vi "JKI SM EDITOR - quick filter list.vi"(0 "quick filter text":string, 1 "Num Event Frames":i32, 7 "States":string[](array[string]), 11 "error in":errorcluster) -> (6 "All Items Filtered Out":bool, 8 "States quick-filtered":string[](array[string]), 10 "Indices quick-filtered":i32[](array[numeric]), 15 "error out":errorcluster)   [LabVIEW 2013]
uses:
  JKI State Machine API/source/JKI SM/JKI SM.lvclass
panel:
  # "Copyright © 2006 James Kring, Inc. All rights reserved.\nMichael Aivaliotis michael.aivaliotis@jameskring.com\nalternate email: michael@aivaliotis.com\n\nThis library is provided \"AS IS\" , WITHOUT WARRANTIES OR \nCONDITIONS OF ANY KIND, either express or implied.\n\nJames Kring, Inc. -- http://www.jameskring.com"
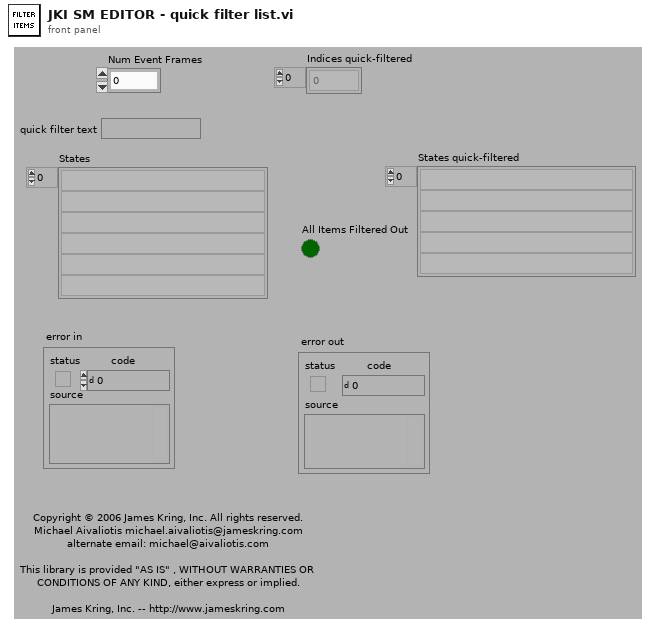
[diagram p1: front panel]
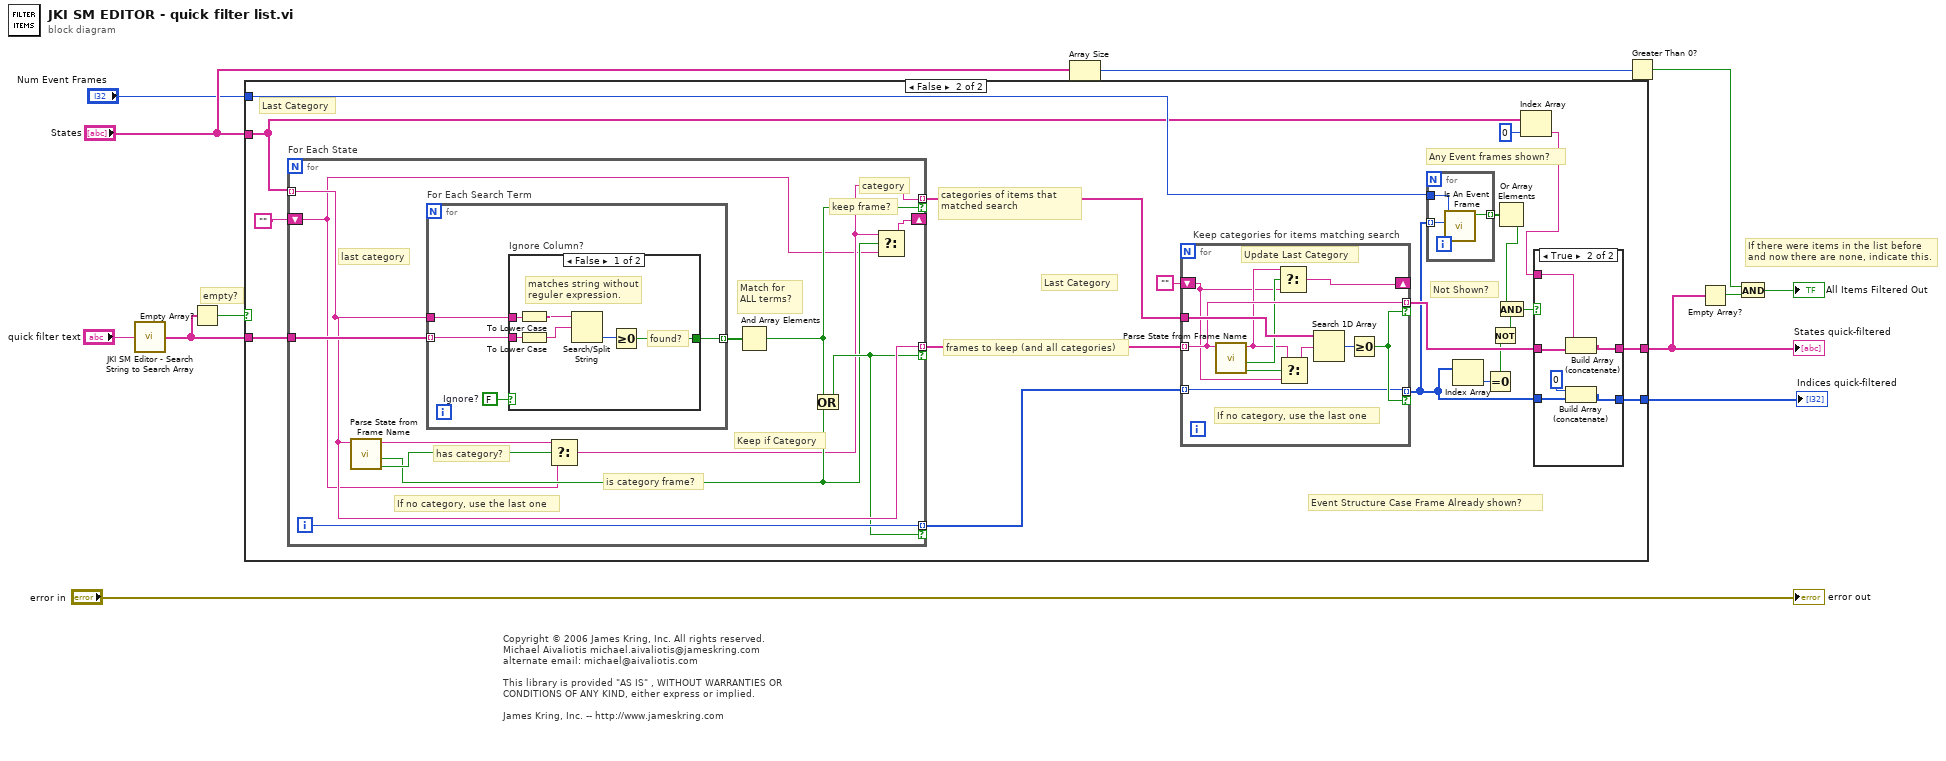
[diagram p0: block diagram]
diagram:
  # "If there were items in the list before and now there are none, indicate this."
  # "Copyright © 2006 James Kring, Inc. All rights reserved.\nMichael Aivaliotis michael.aivaliotis@jameskring.com\nalternate email: michael@aivaliotis.com\n\nThis library is provided \"AS IS\" , WITHOUT WARRANTIES OR \nCONDITIONS OF ANY KIND, either express or implied.\n\nJames Kring, Inc. -- http://www.jameskring.com"
  # "empty?"
  n1 = call "JKI SM Editor - Search String to Search Array.vi"("String"="quick filter text") -> ("Array"=w5:string[])
  n2 = Empty Array?(array=w5) -> (empty?=w4:bool)
  n3 = case shown="False" w4 {
    tunnel: w5 -> [_ w35]
    tunnel: "States" -> [w14 w29]
    tunnel: [w14 w26] -> w11
    tunnel: [w13 w25] -> w2
    tunnel: "Num Event Frames" -> [_ w31]
    frame True {
      # "return previous list untouched."
      n4 = for {
        tunnel: w14 -> [_] mode=indexing
        tunnel: [w15] -> w13 mode=indexing
        i -> [w15]
      }
    }
    frame False {
      # "Last Category"
      # "Last Category"
      # "Any Event frames shown?"
      # "Not Shown?"
      # "Event Structure Case Frame Already shown?"
      # "categories of items that matched search"
      # "frames to keep (and all categories)"
      n5 = for "For Each State" {
        tunnel: w29 -> [w66] mode=indexing
        tunnel: w35 -> [w69]
        tunnel: [w66] -> w32 mode=indexing if=w64
        tunnel: [w59] -> w34 mode=indexing if=w67
        tunnel: [w65] -> w33 mode=indexing if=w64
        shift-right: [w61] -> _
        shift-left: "" -> [w58]
        i -> [w65]
        # "last category"
        # "is category frame?"
        # "If no category, use the last one"
        # "Keep if Category"
        # "category"
        # "keep frame?"
        # "has category?"
        # "Match for ALL terms?"
        n6 = call "Parse State from Frame Name.vi"("Frame or State Name"=w66) -> ("Has Category?"=w63:bool, "is a Category Frame?"=w60:bool, "Category Name"=w62:string)  [unwired: 6 in, 2 out]
        n7 = for "For Each Search Term" {
          tunnel: w66 -> [w73]
          tunnel: w69 -> [w72] mode=indexing
          tunnel: [w71] -> w68 mode=indexing
          w70 = FALSE  # Ignore?
          n8 = case "Ignore Column?" shown="False" w70 {
            tunnel: w73 -> [w79 _]
            tunnel: w72 -> [w78 _]
            tunnel: [w74 _] -> w71
            frame False {
              # "matches string without reguler expression."
              # "found?"
              n9 = To Lower Case(string=w79) -> (all lower case string=w77:string)
              n10 = To Lower Case(string=w78) -> (all lower case string=w76:string)
              n11 = Search/Split String(string=w77, search string/char (-)=w76) -> (offset of match=w75:i32)  [unwired: 1 in, 2 out]
              n12 = Greater Or Equal To 0?(x=w75) -> (x >= 0?=w74:bool)
            }
            frame True {
            }
          }
        }
        n13 = Select(t=w62, s=w63, f=w58) -> (s? t:f=w59:string)
        n14 = And Array Elements(Boolean array=w68) -> (logical AND=w67:bool)
        n15 = Or(x=w67, y=w60) -> (x .or. y?=w64:bool)
        n16 = Select(t=w59, s=w60, f=w58) -> (s? t:f=w61:string)
      }
      n17 = for "Keep categories for items matching search" {
        tunnel: w32 -> [w56] mode=indexing
        tunnel: w34 -> [w57]
        tunnel: [w56] -> w27 mode=indexing if=w54
        tunnel: [w53] -> w23 mode=indexing if=w54
        tunnel: w33 -> [w53] mode=indexing
        shift-right: [w51] -> _
        shift-left: "" -> [w47]
        # "If no category, use the last one"
        # "Update Last Category"
        n18 = call "Parse State from Frame Name.vi"("Frame or State Name"=w56) -> ("Has Category?"=w50:bool, "is a Category Frame?"=w52:bool, "Category Name"=w49:string)  [unwired: 6 in, 2 out]
        n19 = Select(t=w49, s=w52, f=w47) -> (s? t:f=w51:string)
        n20 = Select(t=w49, s=w50, f=w47) -> (s? t:f=w48:string)
        n21 = Search 1D Array(1D array=w57, element=w48) -> (index of element=w55:i32)  [unwired: 1 in]
        n22 = Greater Or Equal To 0?(x=w55) -> (x >= 0?=w54:bool)
      }
      n23 = for {
        tunnel: w23 -> [w46] mode=indexing
        tunnel: w31 -> [w45]
        tunnel: [w44] -> w30 mode=indexing
        n24 = call "Is An Event Frame.vi"("index of element"=w46, "Num Event Frames"=w45) -> ("Event Frame?"=w44:bool)  [unwired: 8 in, 1 out]
      }
      n25 = Index Array(array=w23) -> (element=w22:i32)  [unwired: 1 in]
      n26 = Equal To 0?(x=w22) -> (x = 0?=w21:bool)
      n27 = Not(x=w21) -> (.not. x?=w18:bool)
      n28 = Or Array Elements(Boolean array=w30) -> (logical OR=w20:bool)
      n29 = And(x=w20, y=w18) -> (x .and. y?=w19:bool)
      n30 = Index Array(array=w29, index=0) -> (element=w24:string)
      n31 = case shown="True" w19 {
        tunnel: [w37 w41] -> w26
        tunnel: w27 -> [w37 w42]
        tunnel: [w36 w39] -> w25
        tunnel: w23 -> [w36 w40]
        tunnel: w24 -> [_ w43]
        frame False {
        }
        frame True {
          n32 = Build Array (concatenate)(w43, w42) -> (w41:string[])
          n33 = Build Array (concatenate)(0 ("index"), w40) -> (w39:i32[])
        }
      }
    }
  }
  "States quick-filtered" <- w11
  "Indices quick-filtered" <- w2
  n34 = Array Size(array="States") -> (size(s)=w7:i32)
  n35 = Greater Than 0?(x=w7) -> (x > 0?=w8:bool)
  n36 = Empty Array?(array=w11) -> (empty?=w10:bool)
  n37 = And(x=w8, y=w10) -> (x .and. y?=→"All Items Filtered Out":bool)
  "error out" <- "error in"
